vi "StopRequest.vi"(8 "error in (no error)":errorcluster, 9 "Wait for Module to stop? (F)":bool, 11 "ModuleAdminIn":refnum<class "ModuleAdmin.lvclass">) -> (0 "error out":errorcluster, 2 "Stop Request Sent":bool, 3 "ModuleAdminOut":refnum<class "ModuleAdmin.lvclass">)   [LabVIEW 2018, in "SensorShared.lvlib"]
uses:
  SensorShared.lvlib
  <userlib>/NIST/ModuleAdminLib/ModuleAdmin/ModuleAdmin.lvclass
  <vilib>/event_ctls.llb/usereventprio.ctl
  clStopArgument.ctl
  clEventType.ctl
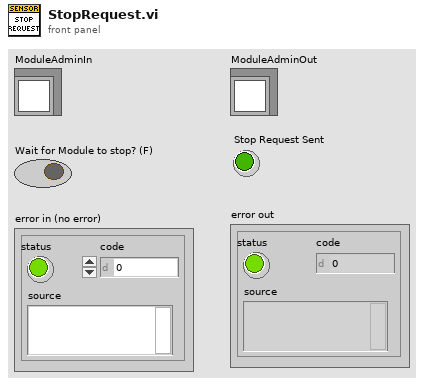
[diagram p1: front panel]
types:
  T1 = typedef "SensorShared.lvlib/clRequestEvents.ctl" = cluster{"StopRequest":refnum<user-event>, "PathToINI":refnum<user-event>, " LoadPlugin":refnum<user-event>, "ShowPanel":refnum<user-event>, "StartData":refnum<user-event>, "StopData":refnum<user-event>, "WriteConfig":refnum<user-event>, "ReadConfig":refnum<user-event>, "WriteEvtSignal":refnum<user-event>, "Configure":refnum<user-event>}
  T2 = typedef "SensorShared.lvlib/clEventType.ctl" = cluster{"ModuleID":i32, "Data":variant}
  T3 = typedef "SensorShared.lvlib/clStopArgument.ctl" = cluster{"Exit via Stop Module Req?":bool, "Wait for Module to stop?":bool, "ModuleAdmin":refnum<class "ModuleAdmin.lvclass">}
  T4 = typedef "usereventprio.ctl" = enum32{"high priority", "normal priority"}
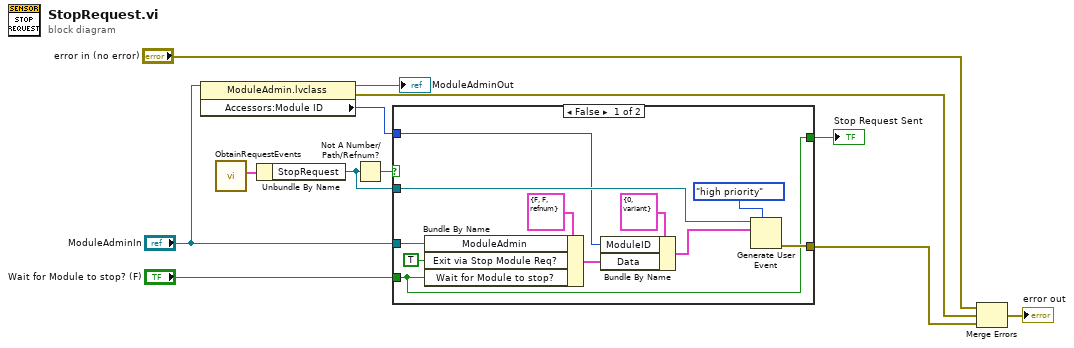
[diagram p0: block diagram]
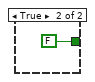
[diagram p2: hidden frame]
diagram:
  n1 = property class="ModuleAdmin.lvclass"(reference="ModuleAdminIn") -> (reference out=→"ModuleAdminOut":refnum<class "ModuleAdmin.lvclass">, error out=w1:errorcluster, "Accessors:Module ID"=w5:i32)  [unwired: 1 in]
  n2 = call "ObtainRequestEvents.vi"() -> ("clRequestEvents"=w12:T1)  [unwired: 10 in, 1 out]
  n3 = Unbundle By Name(w12) -> ("StopRequest"=w10:refnum<user-event>)
  n4 = Not A Number/Path/Refnum?(number/path/refnum=w10) -> (NaN/Path/Refnum?=w11:bool)
  n5 = case shown="False" w11 {
    tunnel: w10 -> [w23 _]
    tunnel: "ModuleAdminIn" -> [w16 _]
    tunnel: "Wait for Module to stop? (F)" -> [w13 _]
    tunnel: [w15 _] -> w7
    tunnel: w5 -> [w14 _]
    tunnel: [w13 FALSE] -> w4
    frame False {
      n6 = Bundle By Name(cluster=T3 {"Exit via Stop Module Req?"=FALSE, "Wait for Module to stop?"=FALSE, "ModuleAdmin"=refnum} ("Stop Argument"), "ModuleAdmin"=w16, "Exit via Stop Module Req?"=TRUE, "Wait for Module to stop?"=w13) -> (w18:T3)
      n7 = Bundle By Name(cluster=T2 {"ModuleID"=0, "Data"=variant} ("clBroadcast"), "ModuleID"=w14, "Data"=w18) -> (w17:T2)
      n8 = Generate User Event(priority (normal)=usereventprio."high priority", user event=w23, event data cluster=w17) -> (error out=w15:errorcluster)  [unwired: 1 in, 1 out]
    }
    frame True {
    }
  }
  "Stop Request Sent" <- w4
  n9 = Merge Errors("error in (no error)", w1, w7) -> (→"error out":errorcluster)
